vi "Write Database.vi"(8 "error in (no error)":errorcluster, 11 "Configuration Database API in":refnum<class "Configuration Database API.lvclass">) -> (0 "error out":errorcluster, 3 "Configuration Database API out":refnum<class "Configuration Database API.lvclass">)   [LabVIEW 2012, in "Configuration Database API.lvlib" / "Configuration Database API.lvclass"]
uses:
  Configuration Database API.lvclass
  Record.ctl
panel:
  in  "Record":T1
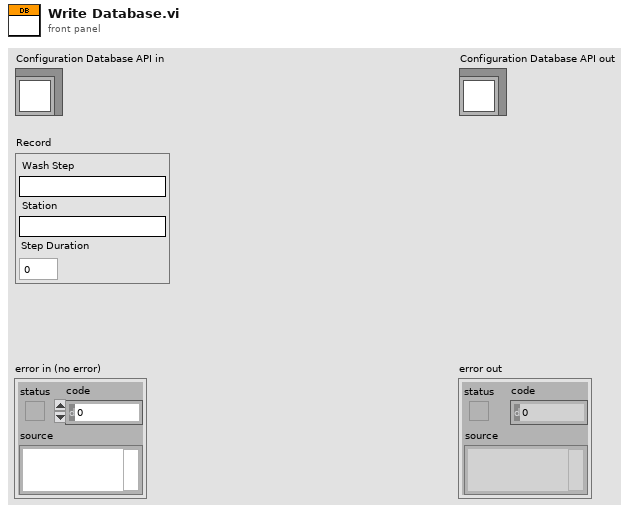
[diagram p1: front panel]
types:
  T1 = typedef "Configuration Database API.lvlib/Configuration Database API.lvclass/Record.ctl" = cluster{"Wash Step":string, "Station":string, "Step Duration":u8}
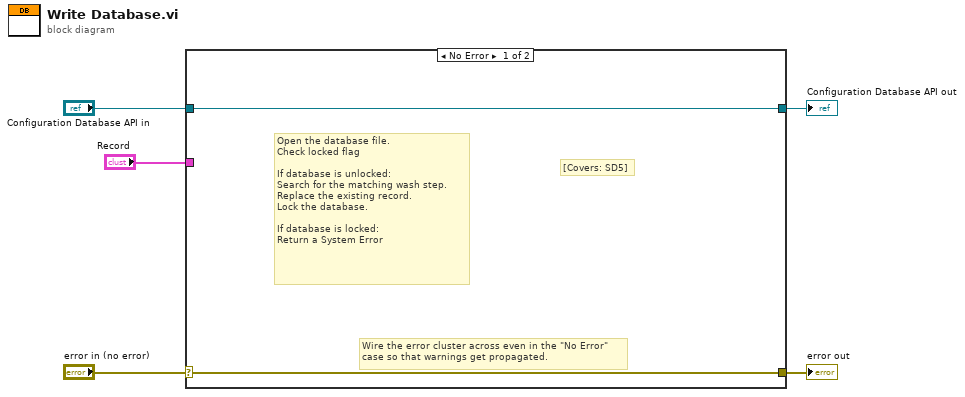
[diagram p0: block diagram]
diagram:
  n1 = case shown="No Error" "error in (no error)" {
    selector: "error in (no error)" -> [w6 w9]
    tunnel: [w6 w9] -> w4
    tunnel: [w7 w8] -> w2
    tunnel: "Configuration Database API in" -> [w7 w8]
    tunnel: "Record" -> [_ _]
    frame No Error {
      # "[Covers: SD5]"
      # "Open the database file.\nCheck locked flag\n\nIf database is unlocked:  \nSearch for the matching wash step.  \nReplace the existing record.\nLock the database.\n\nIf database is locked:\nReturn a System Error"
      # "Wire the error cluster across even in the \"No Error\"\ncase so that warnings get propagated."
    }
    frame Error {
    }
  }
  "error out" <- w4
  "Configuration Database API out" <- w2
